vi "Calc_phase_error.vi"(8 "input valid":bool=TRUE, 11 "Data in":fxp<+/-,16,14>[](array[numeric])=[0.0, 0.0, 0.0, 0.0]) -> (0 "output valid":bool, 3 "Phase error":fxp<+/-,32,4>)   [LabVIEW 2013]
uses:
  <vilib>/rvi/FXPMathLib/FxpAtan2/subVIs/nifxpmath_Atan2_SimConfig.ctl
  <vilib>/rvi/FXPMathLib/FxpAtan2/simVIs/DllFxpAtan2Temp_sub.vi
  <vilib>/rvi/FXPMathLib/FxpAtan2/XNode/nifxpmath_Atan2.xnode
  <vilib>/rvi/FXPMathLib/FxpSub/XNode/nifxpmath_Sub.xnode
  <vilib>/rvi/FXPMathLib/FxpMul/XNode/nifxpmath_Multiplier.xnode
  <vilib>/rvi/FXPMathLib/sim/FxpSim.dll
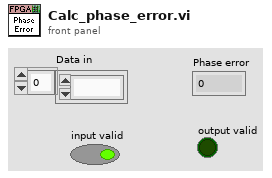
[diagram p1: front panel]
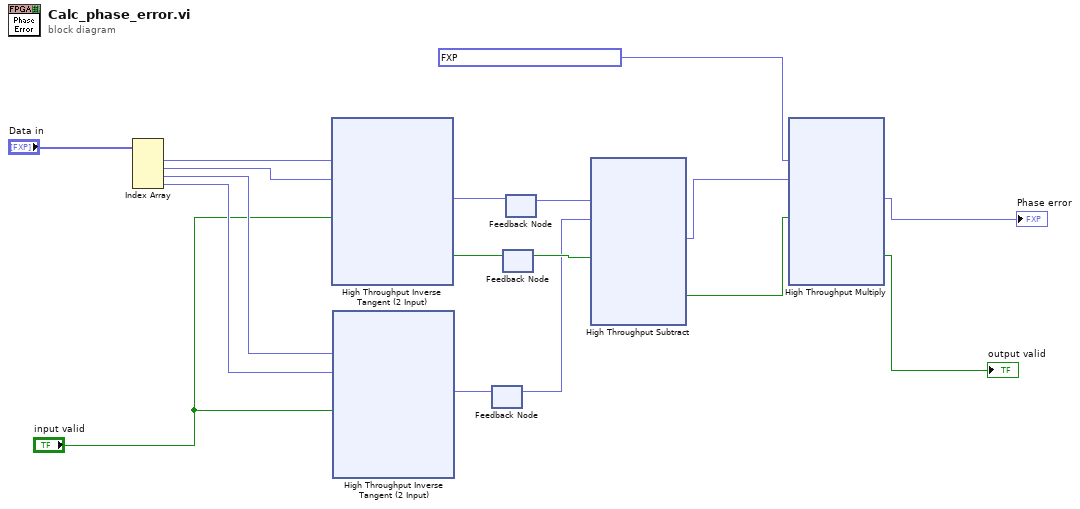
[diagram p0: block diagram]
diagram:
  n1 = Index Array(array="Data in") -> (element #1=w16:fxp<+/-,16,14>, element #2=w15:fxp<+/-,16,14>, element #3=w14:fxp<+/-,16,14>, element #4=w13:fxp<+/-,16,14>)  [unwired: 4 in]
  n2 = xnode "High Throughput Inverse Tangent (2 Input)"("y"=w16, "x"=w15, "input valid"="input valid") -> ("atan2(y,x) (pi)"=w11:fxp<+/-,32,2>, "output valid"=w10:bool)  [unwired: 1 in, 1 out]
  n3 = xnode "High Throughput Inverse Tangent (2 Input)"("y"=w14, "x"=w13, "input valid"="input valid") -> ("atan2(y,x) (pi)"=w8:fxp<+/-,32,2>)  [unwired: 1 in, 2 out]
  n4 = feedback #1() -> (w7:fxp<+/-,32,2>)  [unwired: 1 in]
  n5 = feedback-in #1(w8) -> ()
  n6 = feedback #2() -> (w9:bool)  [unwired: 1 in]
  n7 = feedback-in #2(w10) -> ()
  n8 = feedback #3() -> (w6:fxp<+/-,32,2>)  [unwired: 1 in]
  n9 = feedback-in #3(w11) -> ()
  n10 = xnode "High Throughput Subtract"("x"=w6, "y"=w7, "input valid"=w9) -> ("x-y"=w5:fxp<+/-,32,4>, "output valid"=w3:bool)  [unwired: 1 in, 1 out]
  n11 = xnode ("High Throughput Multiply")("x"=fxp<+/-,32,4> 3.1415926553308964 ("wrap_max"), "y"=w5, "input valid"=w3) -> ("x*y"=→"Phase error":fxp<+/-,32,4>, "output valid"=→"output valid":bool)  [unwired: 1 in, 1 out]
